vi "sub vi - GET ALL TEMP v5.vi"(0 "LA01-EN":bool, 1 "simulate":bool, 5 "LA02-EN":bool, 7 "LA03-EN":bool, 9 "LA04-EN":bool, 11 "LA05-EN":bool, 12 "Gen Cal Value":dbl) -> (4 "LA01 TEMP":T1, 6 "LA02 TEMP":T1, 8 "LA03 TEMP":T1, 10 "LA04 TEMP":T1, 14 "error":bool, 15 "LA05 TEMP":T1)   [LabVIEW 2013]
panel:
  out "LOOP TIME":dbl
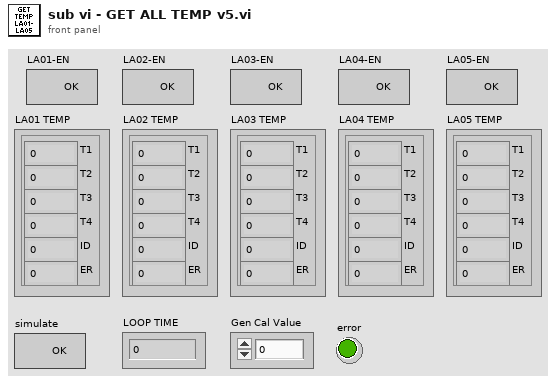
[diagram p1: front panel]
types:
  T1 = cluster{"T1":dbl, "T2":dbl, "T3":dbl, "T4":dbl, "ID":dbl, "ER":dbl}
  T2 = cluster{"T1 Live":dbl, "T1 Neut":dbl, "T2 Live":dbl, "T2 Neut":dbl, "ID":dbl, "ER":dbl}
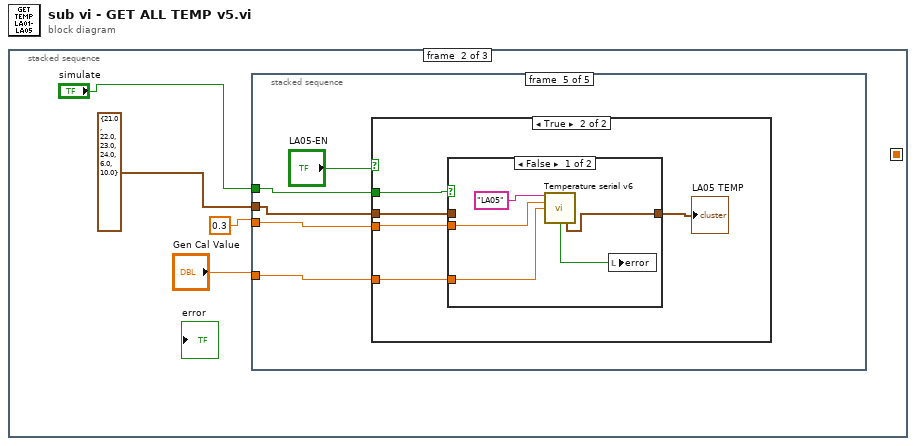
[diagram p0: block diagram]
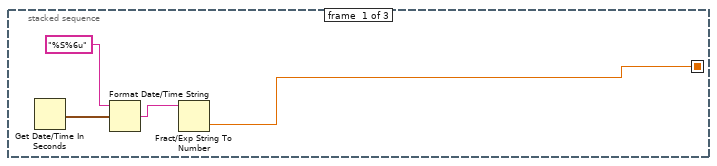
[diagram p2: hidden frame]
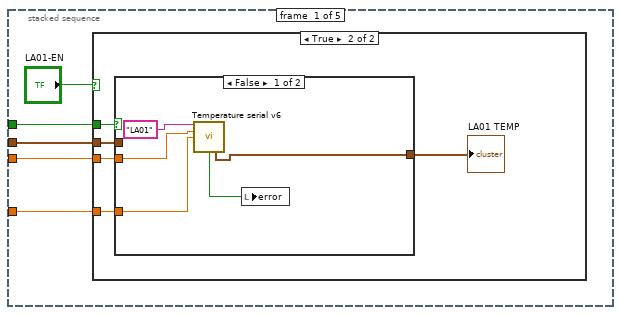
[diagram p3: hidden frame]
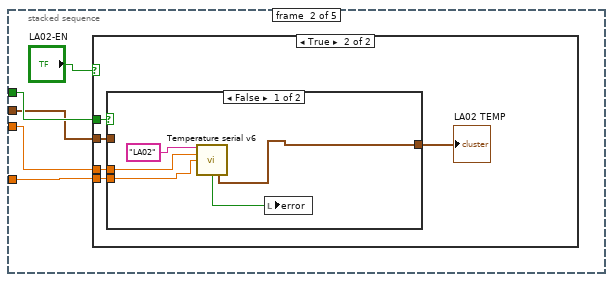
[diagram p6: hidden frame]
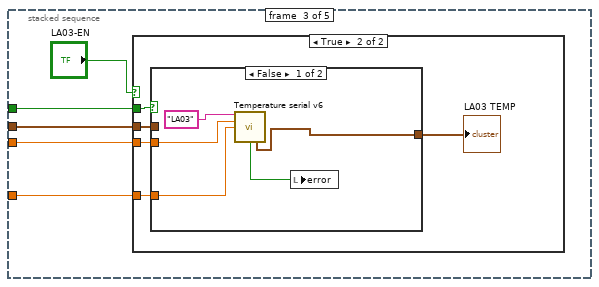
[diagram p9: hidden frame]
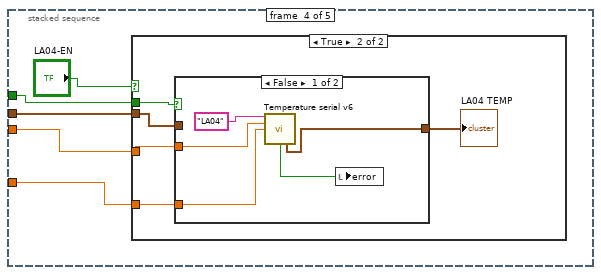
[diagram p12: hidden frame]
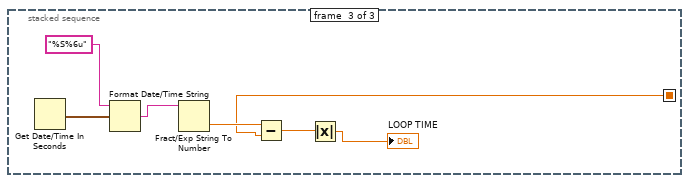
[diagram p17: hidden frame]
diagram:
  n1 = stacked-sequence {
    seq-local: [w1 _ _] -> [_ _ w91]
    frame #0 {
      n2 = Get Date/Time In Seconds() -> (seconds since 1Jan1904=w4:timestamp)
      n3 = Format Date/Time String(time format string (%c)="%S%6u", seconds (now)=w4) -> (date/time string=w2:string)  [unwired: 1 in]
      n4 = Fract/Exp String To Number(string=w2) -> (number=w1:dbl)  [unwired: 3 in, 1 out]
    }
    frame #1 {
      n5 = stacked-sequence {
        tunnel: 0.3 -> [w13 w29 w45 w61 w77]
        tunnel: "Gen Cal Value" -> [w12 w28 w44 w60 w76]
        tunnel: "simulate" -> [w10 w26 w42 w58 w74]
        tunnel: T2 {"T1 Live"=21.0, "T1 Neut"=22.0, "T2 Live"=23.0, "T2 Neut"=24.0, "ID"=6.0, "ER"=10.0} ("LAB01 TEMP") -> [w9 w25 w41 w57 w73]
        frame #0 {
          n6 = case shown="True" "LA01-EN" {
            tunnel: w13 -> [_ w18]
            tunnel: w12 -> [_ w17]
            tunnel: w10 -> [_ w15]
            tunnel: w9 -> [_ w14]
            frame False {
            }
            frame True {
              n7 = case shown="False" w15 {
                tunnel: w18 -> [w22 _]
                tunnel: w17 -> [w21 _]
                tunnel: [w19 w24] -> w16
                tunnel: w14 -> [_ w24]
                frame False {
                  n8 = call "Temperature serial v6.vi"("Command String"="LA01", "Time Out (S)"=w22, "CALIB"=w21) -> ("error"=w20:bool, "output cluster"=w19:cluster{dbl, dbl, dbl, dbl, i32, "error #":dbl})  [unwired: 6 in, 5 out]
                  n9 = local write "error"(w20) -> ()
                }
                frame True {
                }
              }
              "LA01 TEMP" <- w16
            }
          }
        }
        frame #1 {
          n10 = case shown="True" "LA02-EN" {
            tunnel: w29 -> [_ w34]
            tunnel: w28 -> [_ w33]
            tunnel: w26 -> [_ w31]
            tunnel: w25 -> [_ w30]
            frame False {
            }
            frame True {
              n11 = case shown="False" w31 {
                tunnel: w34 -> [w38 _]
                tunnel: w33 -> [w37 _]
                tunnel: [w35 w40] -> w32
                tunnel: w30 -> [_ w40]
                frame False {
                  n12 = call "Temperature serial v6.vi"("Command String"="LA02", "Time Out (S)"=w38, "CALIB"=w37) -> ("error"=w36:bool, "output cluster"=w35:cluster{dbl, dbl, dbl, dbl, i32, "error #":dbl})  [unwired: 6 in, 5 out]
                  n13 = local write "error"(w36) -> ()
                }
                frame True {
                }
              }
              "LA02 TEMP" <- w32
            }
          }
        }
        frame #2 {
          n14 = case shown="True" "LA03-EN" {
            tunnel: w45 -> [_ w50]
            tunnel: w44 -> [_ w49]
            tunnel: w42 -> [_ w47]
            tunnel: w41 -> [_ w46]
            frame False {
            }
            frame True {
              n15 = case shown="False" w47 {
                tunnel: w50 -> [w54 _]
                tunnel: w49 -> [w53 _]
                tunnel: [w51 w56] -> w48
                tunnel: w46 -> [_ w56]
                frame False {
                  n16 = call "Temperature serial v6.vi"("Command String"="LA03", "Time Out (S)"=w54, "CALIB"=w53) -> ("error"=w52:bool, "output cluster"=w51:cluster{dbl, dbl, dbl, dbl, i32, "error #":dbl})  [unwired: 6 in, 5 out]
                  n17 = local write "error"(w52) -> ()
                }
                frame True {
                }
              }
              "LA03 TEMP" <- w48
            }
          }
        }
        frame #3 {
          n18 = case shown="True" "LA04-EN" {
            tunnel: w61 -> [_ w66]
            tunnel: w60 -> [_ w65]
            tunnel: w58 -> [_ w63]
            tunnel: w57 -> [_ w62]
            frame False {
            }
            frame True {
              n19 = case shown="False" w63 {
                tunnel: w66 -> [w70 _]
                tunnel: w65 -> [w69 _]
                tunnel: [w67 w72] -> w64
                tunnel: w62 -> [_ w72]
                frame False {
                  n20 = call "Temperature serial v6.vi"("Command String"="LA04", "Time Out (S)"=w70, "CALIB"=w69) -> ("error"=w68:bool, "output cluster"=w67:cluster{dbl, dbl, dbl, dbl, i32, "error #":dbl})  [unwired: 6 in, 5 out]
                  n21 = local write "error"(w68) -> ()
                }
                frame True {
                }
              }
              "LA04 TEMP" <- w64
            }
          }
        }
        frame #4 {
          n22 = case shown="True" "LA05-EN" {
            tunnel: w77 -> [_ w82]
            tunnel: w76 -> [_ w81]
            tunnel: w74 -> [_ w79]
            tunnel: w73 -> [_ w78]
            frame False {
            }
            frame True {
              n23 = case shown="False" w79 {
                tunnel: w82 -> [w86 _]
                tunnel: w81 -> [w85 _]
                tunnel: [w83 w88] -> w80
                tunnel: w78 -> [_ w88]
                frame False {
                  n24 = call "Temperature serial v6.vi"("Command String"="LA05", "Time Out (S)"=w86, "CALIB"=w85) -> ("error"=w84:bool, "output cluster"=w83:cluster{dbl, dbl, dbl, dbl, i32, "error #":dbl})  [unwired: 6 in, 5 out]
                  n25 = local write "error"(w84) -> ()
                }
                frame True {
                }
              }
              "LA05 TEMP" <- w80
            }
          }
        }
      }
    }
    frame #2 {
      n26 = Get Date/Time In Seconds() -> (seconds since 1Jan1904=w95:timestamp)
      n27 = Format Date/Time String(time format string (%c)="%S%6u", seconds (now)=w95) -> (date/time string=w93:string)  [unwired: 1 in]
      n28 = Fract/Exp String To Number(string=w93) -> (number=w92:dbl)  [unwired: 3 in, 1 out]
      n29 = Subtract(x=w92, y=w91) -> (x-y=w90:dbl)
      n30 = Absolute Value(x=w90) -> (abs(x)=→"LOOP TIME":dbl)
    }
  }
